vi "SessionCfgSave.vi"(8 "error in (no error)":errorcluster, 11 "This VI":refnum<vi>) -> (0 "error out":errorcluster)   [LabVIEW 2019]
uses:
  <vilib>/Utility/config.llb/Write Key (String).vi
  <vilib>/Utility/config.llb/NI_LVConfig.lvlib
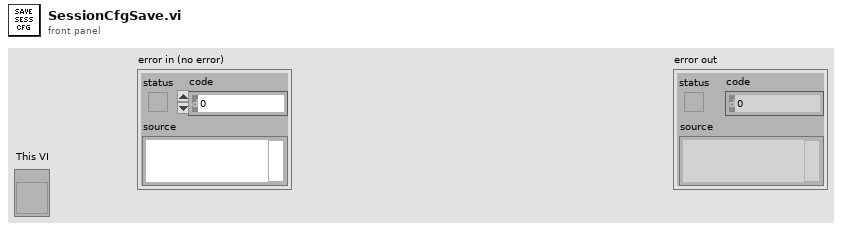
[diagram p1: front panel]
types:
  T1 = typedef "NI_LVConfig.lvlib/Config Data RefNum.ctl" = refnum<k1>
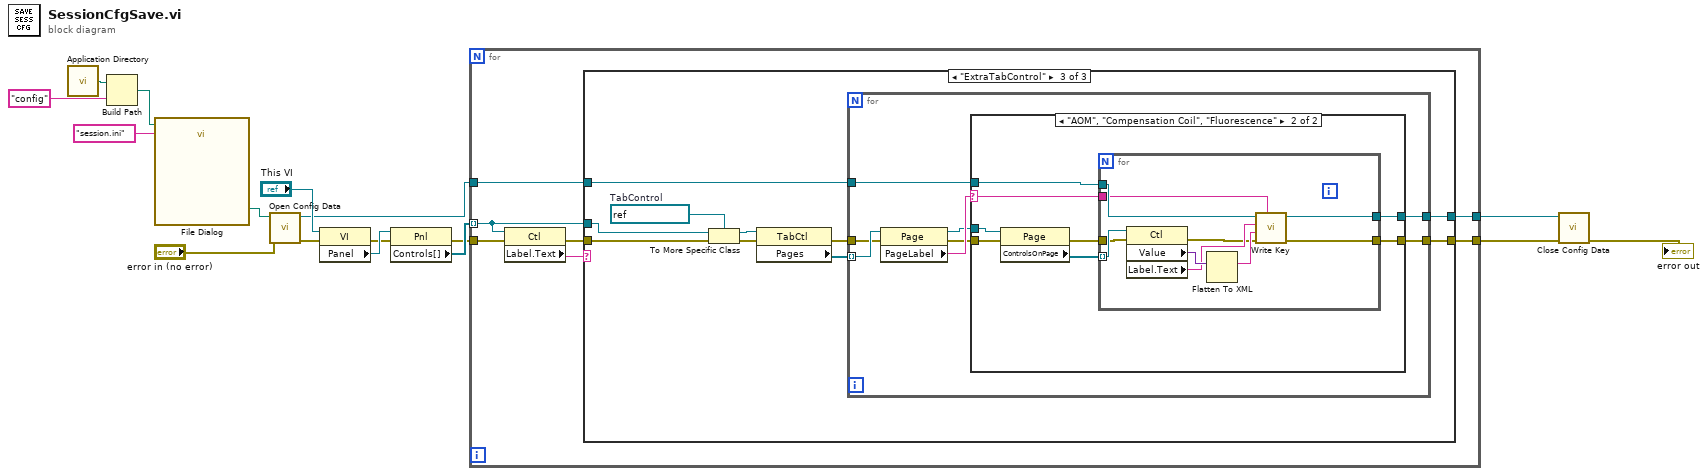
[diagram p0: block diagram]
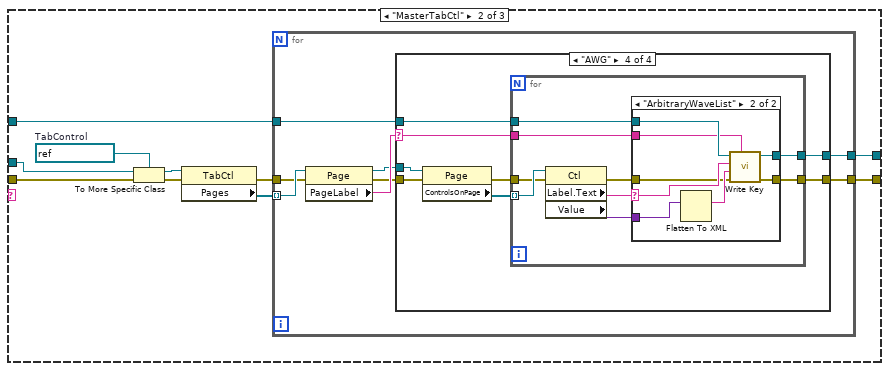
[diagram p3: hidden frame]
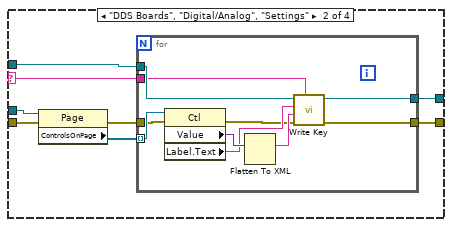
[diagram p5: hidden frame]
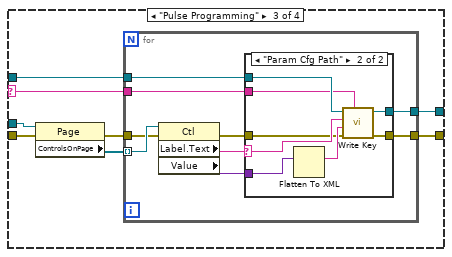
[diagram p6: hidden frame]
diagram:
  n1 = call <vilib>:"Application Directory.vi"() -> ("Application Directory"=w8:path)
  n2 = Build Path(base path=w8, name or relative path="config") -> (appended path=w6:path)
  n3 = call "File Dialog"("start path"=w6, "default name"="session.ini") -> ("selected path"=w10:path)  [unwired: 10 in, 3 out]
  n4 = call <vilib>:"Open Config Data.vi"("error in (no error)"="error in (no error)", "configuration file path"=w10) -> ("error out"=w3:errorcluster, "refnum"=w12:T1)  [unwired: 7 in, 1 out]
  n5 = property class="VI"(reference="This VI", error in=w3) -> (error out=w15:errorcluster, "Panel"=w16:refnum<vi>)  [unwired: 1 out]
  n6 = property class="Pnl"(reference=w16, error in=w15) -> (error out=w5:errorcluster, "Controls[]"=w14:refnum<vi>[])  [unwired: 1 out]
  n7 = for {
    tunnel: w14 -> [w23] mode=indexing
    tunnel: w12 -> [w21]
    tunnel: [w20] -> w11
    tunnel: w5 -> [w19]
    tunnel: [w17] -> w4
    n8 = property class="Ctl"(reference=w23, error in=w19) -> (error out=w18:errorcluster, "Label.Text"=w22:string)  [unwired: 1 out]
    n9 = case shown="\"ExtraTabControl\"" w22 {
      tunnel: w23 -> [_ w32 w124]
      tunnel: w21 -> [w25 w31 w123]
      tunnel: [w25 w30 w122] -> w20
      tunnel: w18 -> [w24 w29 w121]
      tunnel: [w24 w26 w118] -> w17
      frame "False", Default {
      }
      frame "MasterTabCtl" {
        w35 = refnum<vi> refnum  # TabControl
        n10 = To More Specific Class(target class=w35, reference=w32, error in=w29) -> (specific class reference=w34:refnum<vi>, error out=w28:errorcluster)
        n11 = property class="TabCtl"(reference=w34, error in=w28) -> (error out=w27:errorcluster, "Pages"=w33:refnum<vi>[])  [unwired: 1 out]
        n12 = for {
          tunnel: w33 -> [w43] mode=indexing
          tunnel: w31 -> [w40]
          tunnel: [w39] -> w30
          tunnel: w27 -> [w38]
          tunnel: [w36] -> w26
          n13 = property class="Page"(reference=w43, error in=w38) -> (reference out=w41:refnum<vi>, error out=w37:errorcluster, "PageLabel"=w42:string)
          n14 = case shown="\"AWG\"" w42 {
            selector: w42 -> [_ w50 w67 w94]
            tunnel: w41 -> [_ w53 w71 w98]
            tunnel: w40 -> [w45 w51 w69 w96]
            tunnel: [w45 w49 w68 w95] -> w39
            tunnel: w37 -> [w44 w48 w66 w93]
            tunnel: [w44 w46 w64 w91] -> w36
            frame "False", Default {
            }
            frame "DDS Boards", "Digital/Analog", "Settings" {
              n15 = property class="Page"(reference=w53, error in=w48) -> (error out=w47:errorcluster, "ControlsOnPage"=w52:refnum<vi>[])  [unwired: 1 out]
              n16 = for {
                tunnel: w52 -> [w63] mode=indexing
                tunnel: w51 -> [w61]
                tunnel: w50 -> [w60]
                tunnel: [w57] -> w49
                tunnel: w47 -> [w56]
                tunnel: [w54] -> w46
                n17 = property class="Ctl"(reference=w63, error in=w56) -> (error out=w55:errorcluster, "Value"=w62:variant, "Label.Text"=w59:string)  [unwired: 1 out]
                n18 = Flatten To XML(anything=w62) -> (xml string=w58:string)
                n19 = call-poly <vilib>:"Write Key.vi"("section"=w60, "error in (no error)"=w55, "value"=w58, "key"=w59, "refnum"=w61) -> ("error out"=w54:errorcluster, "refnum out"=w57:T1)  [unwired: 4 in, 1 out]
              }
            }
            frame "Pulse Programming" {
              n20 = property class="Page"(reference=w71, error in=w66) -> (error out=w65:errorcluster, "ControlsOnPage"=w70:refnum<vi>[])  [unwired: 1 out]
              n21 = for {
                tunnel: w70 -> [w80] mode=indexing
                tunnel: w69 -> [w77]
                tunnel: [w76] -> w68
                tunnel: w67 -> [w75]
                tunnel: w65 -> [w74]
                tunnel: [w72] -> w64
                n22 = property class="Ctl"(reference=w80, error in=w74) -> (error out=w73:errorcluster, "Label.Text"=w79:string, "Value"=w78:variant)  [unwired: 1 out]
                n23 = case shown="\"Param Cfg Path\"" w79 {
                  selector: w79 -> [_ w86]
                  tunnel: w78 -> [_ w89]
                  tunnel: w77 -> [w82 w88]
                  tunnel: [w82 w87] -> w76
                  tunnel: w75 -> [_ w85]
                  tunnel: w73 -> [w81 w84]
                  tunnel: [w81 w83] -> w72
                  frame "False", Default {
                  }
                  frame "Param Cfg Path" {
                    n24 = Flatten To XML(anything=w89) -> (xml string=w90:string)
                    n25 = call-poly <vilib>:"Write Key.vi"("section"=w85, "error in (no error)"=w84, "value"=w90, "key"=w86, "refnum"=w88) -> ("error out"=w83:errorcluster, "refnum out"=w87:T1)  [unwired: 4 in, 1 out]
                  }
                }
              }
            }
            frame "AWG" {
              n26 = property class="Page"(reference=w98, error in=w93) -> (error out=w92:errorcluster, "ControlsOnPage"=w97:refnum<vi>[])  [unwired: 1 out]
              n27 = for {
                tunnel: w97 -> [w107] mode=indexing
                tunnel: w96 -> [w104]
                tunnel: [w103] -> w95
                tunnel: w94 -> [w102]
                tunnel: w92 -> [w101]
                tunnel: [w99] -> w91
                n28 = property class="Ctl"(reference=w107, error in=w101) -> (error out=w100:errorcluster, "Label.Text"=w106:string, "Value"=w105:variant)  [unwired: 1 out]
                n29 = case shown="\"ArbitraryWaveList\"" w106 {
                  selector: w106 -> [_ w113]
                  tunnel: w105 -> [_ w116]
                  tunnel: w104 -> [w109 w115]
                  tunnel: [w109 w114] -> w103
                  tunnel: w102 -> [_ w112]
                  tunnel: w100 -> [w108 w111]
                  tunnel: [w108 w110] -> w99
                  frame "False", Default {
                  }
                  frame "ArbitraryWaveList" {
                    n30 = Flatten To XML(anything=w116) -> (xml string=w117:string)
                    n31 = call-poly <vilib>:"Write Key.vi"("section"=w112, "error in (no error)"=w111, "value"=w117, "key"=w113, "refnum"=w115) -> ("error out"=w110:errorcluster, "refnum out"=w114:T1)  [unwired: 4 in, 1 out]
                  }
                }
              }
            }
          }
        }
      }
      frame "ExtraTabControl" {
        w127 = refnum<vi> refnum  # TabControl
        n32 = To More Specific Class(target class=w127, reference=w124, error in=w121) -> (specific class reference=w126:refnum<vi>, error out=w120:errorcluster)
        n33 = property class="TabCtl"(reference=w126, error in=w120) -> (error out=w119:errorcluster, "Pages"=w125:refnum<vi>[])  [unwired: 1 out]
        n34 = for {
          tunnel: w125 -> [w135] mode=indexing
          tunnel: w123 -> [w132]
          tunnel: [w131] -> w122
          tunnel: w119 -> [w130]
          tunnel: [w128] -> w118
          n35 = property class="Page"(reference=w135, error in=w130) -> (reference out=w133:refnum<vi>, error out=w129:errorcluster, "PageLabel"=w134:string)
          n36 = case shown="\"AOM\", \"Compensation Coil\", \"Fluorescence\"" w134 {
            selector: w134 -> [_ w142]
            tunnel: w133 -> [_ w145]
            tunnel: w132 -> [w137 w143]
            tunnel: [w137 w141] -> w131
            tunnel: w129 -> [w136 w140]
            tunnel: [w136 w138] -> w128
            frame "False", Default {
            }
            frame "AOM", "Compensation Coil", "Fluorescence" {
              n37 = property class="Page"(reference=w145, error in=w140) -> (error out=w139:errorcluster, "ControlsOnPage"=w144:refnum<vi>[])  [unwired: 1 out]
              n38 = for {
                tunnel: w144 -> [w155] mode=indexing
                tunnel: w143 -> [w153]
                tunnel: w142 -> [w152]
                tunnel: [w149] -> w141
                tunnel: w139 -> [w148]
                tunnel: [w146] -> w138
                n39 = property class="Ctl"(reference=w155, error in=w148) -> (error out=w147:errorcluster, "Value"=w154:variant, "Label.Text"=w151:string)  [unwired: 1 out]
                n40 = Flatten To XML(anything=w154) -> (xml string=w150:string)
                n41 = call-poly <vilib>:"Write Key.vi"("section"=w152, "error in (no error)"=w147, "value"=w150, "key"=w151, "refnum"=w153) -> ("error out"=w146:errorcluster, "refnum out"=w149:T1)  [unwired: 4 in, 1 out]
              }
            }
          }
        }
      }
    }
  }
  n42 = call <vilib>:"Close Config Data.vi"("error in (no error)"=w4, "refnum"=w11) -> ("error out"=→"error out":errorcluster)  [unwired: 8 in, 1 out]
